vi "_Remote Prepare Run 2 Data.vi"(6 "error in":errorcluster) -> (0 "error out":errorcluster, 1 "Steps":i32[][](array[numeric]), 2 "Scans":i32, 3 "Mass":dbl[][](array[numeric]), 4 "AcqMethod":T1[](array[typedef]) {"ScanType" format="%#.6g"; "Mass Range"."Res" items=["High/High", "Medium/Medium", "Low/Low", "High/Medium", "High/Low", "Medium/High", "Medium/Low", "Low/High", "Low/Medium"]}, 5 "Dwell":dbl[][](array[numeric]))   [LabVIEW 2015]
uses:
  Type/_XML Expt.ctl
  Type/_XML Lens.ctl
  Type/_Mass Range Property.ctl
  Type/_Mass Range Parameters.ctl
  Type/_RT Res Type.ctl
  Type/_RT Parameter.ctl
  Type/_RT Active Ch.ctl
  Type/_RT Expt.ctl
  Type/_Run Mode.ctl
  Type/_RT Mass Range.ctl
  Type/_RT Command.ctl
  Configuration/_Global Configuration.vi
panel:
  # "(# of Expts) X (# of Masses)"
  # "(# of Expts) X (# of MassRanges)"
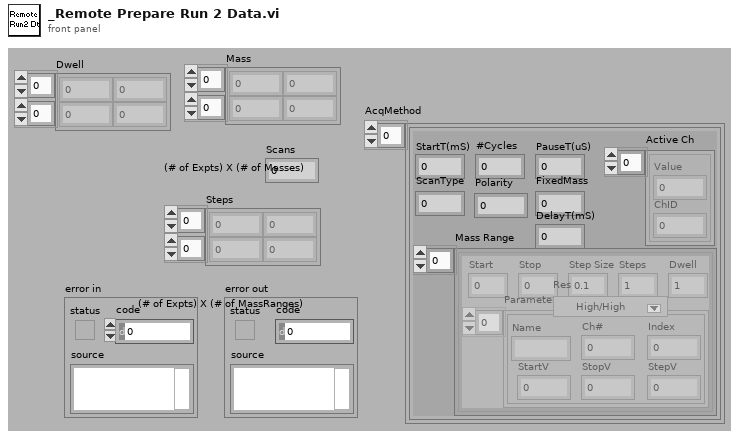
[diagram p1: front panel]
types:
  T1 = typedef "_XML Expt.ctl" = cluster{"StartT(mS)":i32, "#Cycles":i32, "PauseT(uS)":i32, "ScanType":i32, "Polarity":u8, "FixedMass":dbl, "DelayT(mS)":i32, "Active Ch":T2[], "Mass Range":T3[]}
  T2 = typedef "_XML Lens.ctl" = cluster{"Value":dbl, "ChID":u8}
  T3 = typedef "_Mass Range Property.ctl" = cluster{"Start":dbl, "Stop":dbl, "Step Size":dbl, "Steps":i32, "Dwell":dbl, "Parameters":T4[], "Res":T5}
  T4 = typedef "_Mass Range Parameters.ctl" = cluster{"Name":string, "Ch#":u8, "StartV":dbl, "StopV":dbl, "StepV":dbl, "Index":u8}
  T5 = typedef "_RT Res Type.ctl" = u16
  T6 = typedef "_RT Command.ctl" = enum16{"Start", "StartActualRun", "Stop", "Runtime Update", "Get Data", "Get Info", "Get Status", "Get Param", "Get Config", "Get Table", "Read ADC", "Set Oscillator", "Update Config", "Update Table", "Set All Pol", "Set Pol and DC", "Set Max Mass", "Toggle RP", "Toggle EL", "Set PIC", "Initialize Turbo", "Send Turbo Comm", "Close Turbo", "P1", "P2", "P3", "Send Serial", "Set LC Out", "Get LC In", "Read VAC", "Test Table", "Toggle Power", "Get Startup", "Set Startup", "Get ADC Table", "Set ADC Table", "Get Brief Status", "Get Detail Status", "Auxiliary Update", "Set CC Logics", "Set CC Input Logics", "Ignore Error"}
  T7 = typedef "_RT Active Ch.ctl" = cluster{"Start":i32, "Step":i32, "ChID":i32}
  T8 = typedef "_RT Expt.ctl" = cluster{"StartT(mS)":i32, "#Cycles":i32, "Scan Type":T9, "PauseT(uS)":i32, "Polarity":u8, "DelayT(mS)":i32, "Active Ch":T7[], "Mass Range":T10[]}
  T9 = typedef "_Run Mode.ctl" = enum16{"MRM (Q1/Q2)", "Q1 Scan", "Q1 SRM", "Q2 Scan", "Q2 SRM", "Product Scan", "Precursor Scan", "Neutral Loss", "Neutral Gain"}
  T10 = typedef "_RT Mass Range.ctl" = cluster{"Steps":i32, "Dwell(uS)":i32, "Resolution Type":T5, "Ramping Ch":T7[]}
  T11 = typedef "_RT Parameter.ctl" = cluster{"RunMode":i32, "Initial Ch":T7[], "Sync":u8, "Expt":T8[], "EqTime(mS)":i32}
  T12 = typedef "_Lens Property.ctl" = cluster{"Scan Type":u8, "Scans":i32, "Time 1":dbl, "Time 2":dbl, "Value 1":dbl, "Value 2":dbl, "Step Size":dbl}
  T13 = cluster{"Lenses":T12[], "Mass Ranges":T3[], "Acquire":bool, "MCA":bool, "Q1DC EN":bool, "Q1 POL":bool, "Q3 POL":bool, "Q1 RF  EN":bool, "Averaging":bool, "Log Scale":bool, "CPS":bool, "Unit":bool, "Data Path":path, "Run Mode":T9, "Fixed Mass (amu)":dbl, "Q3DC EN":bool, "Q3 RF  EN":bool, "Negative":bool}
  T14 = typedef "_RT Instrument 2.ctl" = cluster{"Table":T15[], "Instrument":string[]}
  T15 = typedef "_RT Configuration 2.ctl" = cluster{"Name":string, "Ch#":u8, "Min":dbl, "Max":dbl, "Def+":dbl, "Def-":dbl, "Offset":dbl, "Slope":dbl, "Type":u8, "Description":string, "SettleT":dbl}
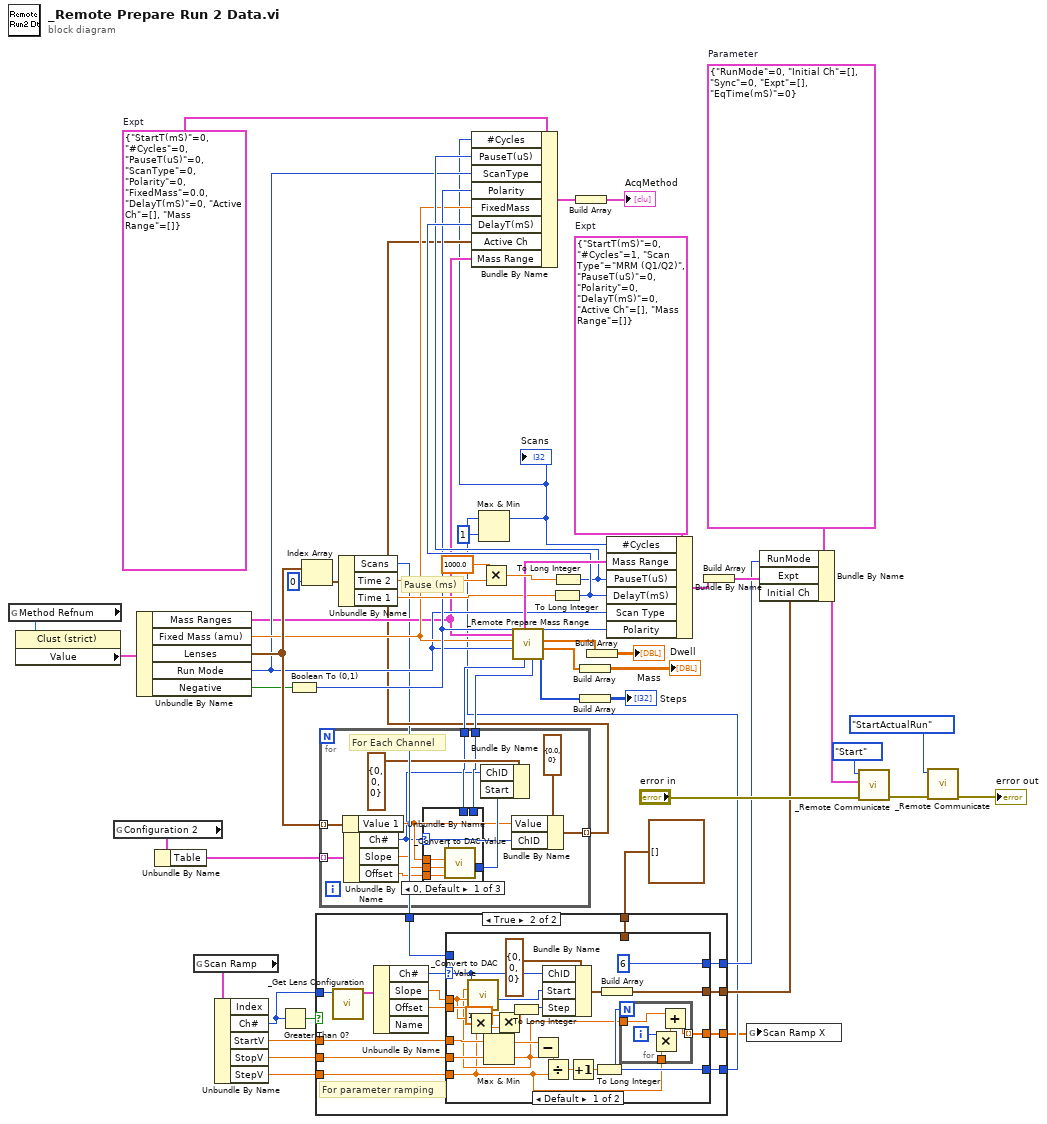
[diagram p0: block diagram]
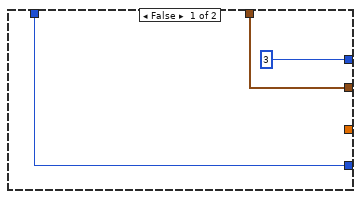
[diagram p2: hidden frame]
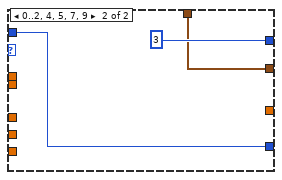
[diagram p3: hidden frame]
diagram:
  w29 = T1 {"StartT(mS)"=0, "#Cycles"=0, "PauseT(uS)"=0, "ScanType"=0, "Polarity"=0, "FixedMass"=0.0, "DelayT(mS)"=0, "Active Ch"=[], "Mass Range"=[]}  # Expt
  w54 = T8 {"StartT(mS)"=0, "#Cycles"=1, "Scan Type"=enum."MRM (Q1/Q2)", "PauseT(uS)"=0, "Polarity"=0, "DelayT(mS)"=0, "Active Ch"=[], "Mass Range"=[]}  # Expt
  w55 = T11 {"RunMode"=0, "Initial Ch"=[], "Sync"=0, "Expt"=[], "EqTime(mS)"=0}  # Parameter
  # "Pause (ms)"
  n1 = global read "_Global Configuration.vi" "Method Refnum"() -> (w49:refnum<vi>)
  n2 = property class="Clust (strict)"(reference=w49) -> ("Value"=w47:T13)  [unwired: 1 in, 2 out]
  n3 = global read "_Global Configuration.vi" "Configuration 2"() -> (w48:T14)
  n4 = Unbundle By Name(w47) -> ("Mass Ranges"=w21:T3[], "Fixed Mass (amu)"=w23:dbl, "Lenses"=w35:T12[], "Run Mode"=w22:T9, "Negative"=w31:bool)
  n5 = Unbundle By Name(w48) -> ("Table"=w39:T15[])
  n6 = global read "_Global Configuration.vi" "Scan Ramp"() -> (w17:T4)
  n7 = Unbundle By Name(w17) -> ("Ch#"=w12:u8, "StartV"=w16:dbl, "StopV"=w15:dbl, "StepV"=w13:dbl)  [unwired: 1 out]
  n8 = Greater Than 0?(x=w12) -> (x > 0?=w14:bool)
  n9 = Boolean To (0,1)(Boolean=w31) -> (0, 1=w24:i16)
  n10 = Index Array(array=w35, index=0) -> (element=w44:T12)
  n11 = Unbundle By Name(w44) -> ("Scans"=w9:i32, "Time 2"=w42:dbl, "Time 1"=w30:dbl)
  n12 = case shown="True" w14 {
    tunnel: w16 -> [_ w68]
    tunnel: w15 -> [_ w66]
    tunnel: w13 -> [_ w61]
    tunnel: w12 -> [_ w71]
    tunnel: w9 -> [w57 w65]
    tunnel: [w56 w64] -> w11
    tunnel: T7[] [] ("Active Ch") -> [w56 w63]
    tunnel: [3 ("RunMode") w62] -> w10
    tunnel: [w57 w60] -> w8
    tunnel: [_ w59] -> w5
    frame False {
    }
    frame True {
      # "For parameter ramping"
      n13 = call "_Get Lens Configuration.vi"("Channel #"=w71) -> ("Lens Configuration"=w72:T15)  [unwired: 1 in, 5 out]
      n14 = Unbundle By Name(w72) -> ("Ch#"=w67:u8, "Slope"=w70:dbl, "Offset"=w69:dbl)  [unwired: 1 out]
      n15 = case shown="Default" w67 {
        selector: w67 -> [w91 _]
        tunnel: w70 -> [w93 _]
        tunnel: w69 -> [w94 _]
        tunnel: w68 -> [w81 _]
        tunnel: w66 -> [w82 _]
        tunnel: w65 -> [_ w101]
        tunnel: [w87 w100] -> w64
        tunnel: w63 -> [_ w100]
        tunnel: [6 ("RunMode") 3 ("RunMode")] -> w62
        tunnel: w61 -> [w77 _]
        tunnel: [w79 w101] -> w60
        tunnel: [w76 _] -> w59
        frame Default {
          n16 = Multiply(x=w93, y=w77) -> (x*y=w75:dbl)
          n17 = Max & Min(x=w81, y=w82) -> (max(x,y)=w85:dbl, min(x,y)=w78:dbl)
          n18 = call "_Convert to DAC Value.vi"("Offset"=w94, "Slop"=w93, "Number"=w78, "Channel"=w91) -> ("DAC Value"=w90:i32)  [unwired: 2 in, 5 out]
          n19 = Multiply(x=128.0, y=w75) -> (x*y=w74:dbl)
          n20 = To Long Integer(number=w74) -> (32bit integer=w89:i32)
          n21 = Subtract(x=w85, y=w78) -> (x-y=w84:dbl)
          n22 = Bundle By Name(cluster=T7 {"Start"=0, "Step"=0, "ChID"=0} ("Active Channel"), "ChID"=w91, "Start"=w90, "Step"=w89) -> (w88:T7)
          n23 = Divide(x=w84, y=w77) -> (x/y=w83:dbl)
          n24 = Increment(x=w83) -> (x+1=w80:dbl)
          n25 = To Long Integer(number=w80) -> (32bit integer=w79:i32)
          n26 = Build Array(w88) -> (w87:T7[])
          n27 = for {
            N: w79 -> [_]
            tunnel: w78 -> [w97]
            tunnel: [w96] -> w76 mode=indexing
            tunnel: w77 -> [w95]
            i -> [w99]
            n28 = Multiply(x=w99, y=w95) -> (x*y=w98:dbl)
            n29 = Add(x=w97, y=w98) -> (x+y=w96:dbl)
          }
        }
        frame 0..2, 4, 5, 7, 9 {
        }
      }
    }
  }
  n30 = Max & Min(x=w8, y=1) -> (max(x,y)=w19:i32)  [unwired: 1 out]
  "Scans" <- w19
  n31 = Multiply(x=1000.0 ("y"), y=w42) -> (x*y=w43:dbl)
  n32 = call "_Remote Prepare Mass Range.vi"("Run Mode"=w22, "Fixed Mass (amu)"=w23, "GUI Mass Ranges"=w21) -> ("Steps"=w37:i32[], "Dwell (ms)"=w36:dbl[], "Mass"=w6:dbl[], "Init Q2 Mass"=w33:i32, "Init Q1 Mass"=w34:i32, "RT Mass Ranges"=w38:T10[])  [unwired: 3 out]
  n33 = for {
    tunnel: w39 -> [w110] mode=indexing
    tunnel: w35 -> [w109] mode=indexing
    tunnel: w34 -> [w108]
    tunnel: w33 -> [w107]
    tunnel: [w103] -> w20 mode=indexing
    # "For Each Channel"
    n34 = Unbundle By Name(w109) -> ("Value 1"=w105:dbl)
    n35 = Unbundle By Name(w110) -> ("Ch#"=w104:u8, "Slope"=w114:dbl, "Offset"=w113:dbl)
    n36 = case shown="0, Default" w104 {
      selector: w104 -> [w115 _ _]
      tunnel: w105 -> [w119 _ _]
      tunnel: w114 -> [w118 _ _]
      tunnel: w113 -> [w117 _ _]
      tunnel: [w116 w120 w121] -> w111
      tunnel: w108 -> [_ w120 _]
      tunnel: w107 -> [_ _ w121]
      frame 0, Default {
        n37 = call "_Convert to DAC Value.vi"("Offset"=w117, "Slop"=w118, "Number"=w119, "Channel"=w115) -> ("DAC Value"=w116:i32)  [unwired: 2 in, 5 out]
      }
      frame 1, 4, 7 {
        # "for Q1"
      }
      frame 2, 5, 9 {
        # "for Q3"
      }
    }
    n38 = Bundle By Name(cluster=T7 {"Start"=0, "Step"=0, "ChID"=0} ("Active Channel"), "ChID"=w104, "Start"=w111) -> ()  [unwired: 1 out]
    n39 = Bundle By Name(cluster=T2 {"Value"=0.0, "ChID"=0} ("Lens"), "Value"=w105, "ChID"=w104) -> (w103:T2)
  }
  n40 = To Long Integer(number=w30) -> (32bit integer=w26:i32)
  n41 = To Long Integer(number=w43) -> (32bit integer=w25:i32)
  n42 = Bundle By Name(cluster=w29, "#Cycles"=w19, "PauseT(uS)"=w25, "ScanType"=w22, "Polarity"=w24, "FixedMass"=w23, "DelayT(mS)"=w26, "Active Ch"=w20, "Mass Range"=w21) -> (w28:T1)
  n43 = Build Array(w28) -> (→"AcqMethod":T1[])
  n44 = Build Array(w36) -> (→"Dwell":dbl[][])
  n45 = Build Array(w37) -> (→"Steps":i32[][])
  n46 = Build Array(w6) -> (→"Mass":dbl[][])
  n47 = Bundle By Name(cluster=w54, "#Cycles"=w19, "Mass Range"=w38, "PauseT(uS)"=w25, "DelayT(mS)"=w26, "Scan Type"=w22, "Polarity"=w24) -> (w53:T8)
  n48 = Build Array(w53) -> (w52:T8[])
  n49 = global write "_Global Configuration.vi" "Scan Ramp X"(w5) -> ()
  n50 = Bundle By Name(cluster=w55, "RunMode"=w10, "Expt"=w52, "Initial Ch"=w11) -> (w51:T11)
  n51 = call "_Remote Communicate.vi"("error in (no error)"="error in", "Parameter"=w51, "Command"=_RT_Command."Start") -> ("error out"=w1:errorcluster)  [unwired: 3 in, 3 out]
  n52 = call "_Remote Communicate.vi"("error in (no error)"=w1, "Command"=_RT_Command."StartActualRun") -> ("error out"=→"error out":errorcluster)  [unwired: 4 in, 3 out]
